vi "indicator.vi"() -> ()   [LabVIEW 2009]
panel:
  in  "stop":bool
  out "Waveform Chart":i32(graph)
  out "Numeric":i32
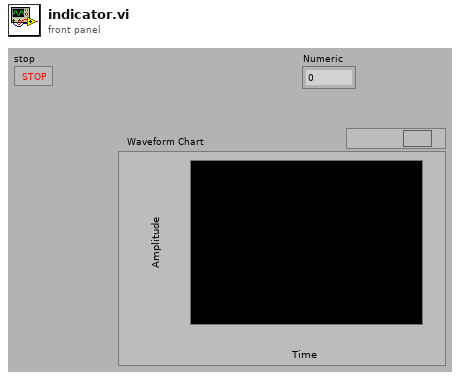
[diagram p1: front panel]
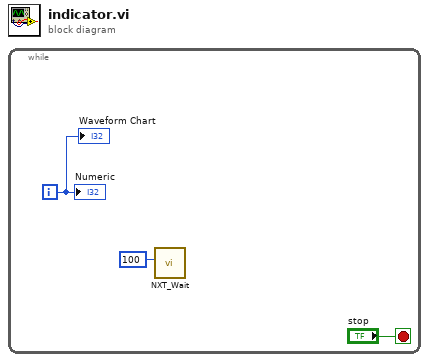
[diagram p0: block diagram]
diagram:
  n1 = while {
    i -> [w2]
    stop <- "stop" stop-if-true
    n2 = call <vilib>:"NXT_Wait.vi"("Wait (ms)"=u32 100) -> ()  [unwired: 9 in, 2 out]
    "Numeric" <- w2
    "Waveform Chart" <- w2
  }
